vi "NF WF1973_74 INST Coup.vi"(6 "Read(F)":bool, 8 "error in (no error)":errorcluster caption="Error IN", 10 "Couple(None)":u16(ring)=1 items=["All", "None"], 11 "VISAsession":refnum<visa-resource-name>) -> (0 "error out":errorcluster caption="Error OUT", 2 "Query Mode":string, 3 "CopyVISAsession":refnum<visa-resource-name>)   [LabVIEW 2010]
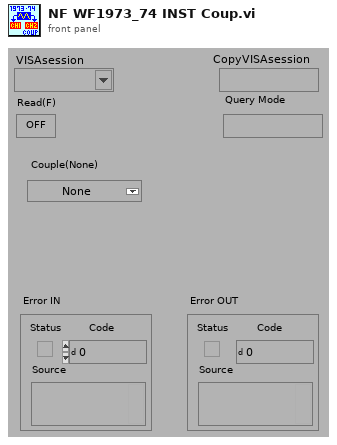
[diagram p1: front panel]
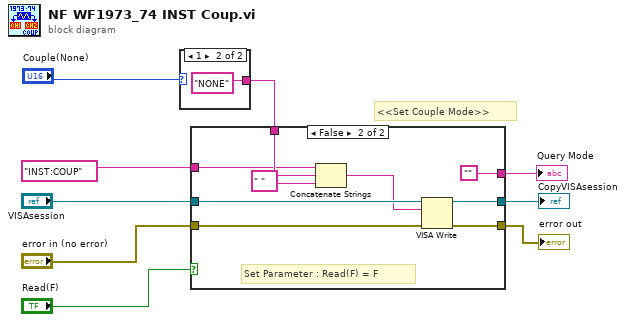
[diagram p0: block diagram]
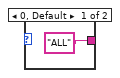
[diagram p2: hidden frame]
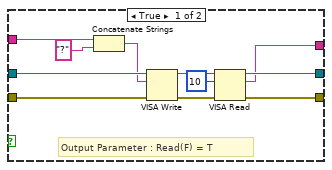
[diagram p3: hidden frame]
diagram:
  # "<<Set Couple Mode>>"
  n1 = case shown="1" "Couple(None)" {
    tunnel: ["ALL" ("文字列") "NONE" ("文字列")] -> w1
    frame 0, Default {
    }
    frame 1 {
    }
  }
  n2 = case shown="FALSE" "Read(F)" {
    tunnel: "VISAsession" -> [w22 w31]
    tunnel: [w19 w28] -> w8
    tunnel: [w18 w29] -> w7
    tunnel: "error in (no error)" -> [w17 w30]
    tunnel: "INST:COUP" ("文字列") -> [w15 w23]
    tunnel: [w12 ""] -> w3
    tunnel: w1 -> [_ w25]
    frame True {
      # "Output Parameter : Read(F) = T"
      n3 = Concatenate Strings(w15, "?" ("形式文字列")) -> (w13:string)
      n4 = VISA Write(VISA resource name=w22, write buffer=w13, error in (no error)=w17) -> (VISA resource name out=w20:refnum<visa-resource-name>, error out=w21:errorcluster)  [unwired: 1 out]
      n5 = VISA Read(VISA resource name=w20, byte count=u32 10 ("バイトカウント（0）"), error in (no error)=w21) -> (VISA resource name out=w19:refnum<visa-resource-name>, read buffer=w12:string, error out=w18:errorcluster)  [unwired: 1 out]
    }
    frame False {
      # "Set Parameter : Read(F) = F"
      n6 = Concatenate Strings(w23, " ", w25) -> (w26:string)
      n7 = VISA Write(VISA resource name=w31, write buffer=w26, error in (no error)=w30) -> (VISA resource name out=w28:refnum<visa-resource-name>, error out=w29:errorcluster)  [unwired: 1 out]
    }
  }
  "error out" <- w7
  "CopyVISAsession" <- w8
  "Query Mode" <- w3
